vi "Sort Section Nodes.vi"(8 "error in":errorcluster, 10 "Nested Section Types":cluster{"Nested Section Types":string[]}[](array[cluster]), 11 "Section TypeNames":string[](array[string])) -> (0 "error out":errorcluster, 3 "Sorted Section TypeNames":string[](array[string]))   [LabVIEW 2026, in "Plugin XML Parser.lvlib"]
uses:
  Plugin XML Parser.lvlib
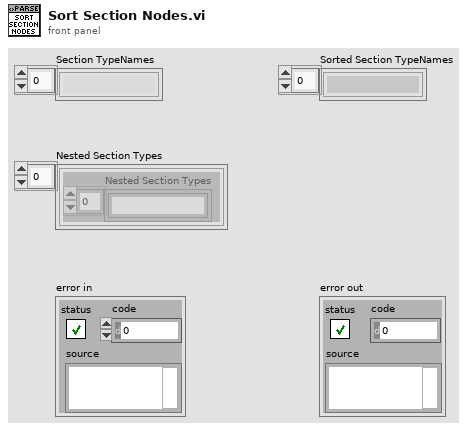
[diagram p1: front panel]
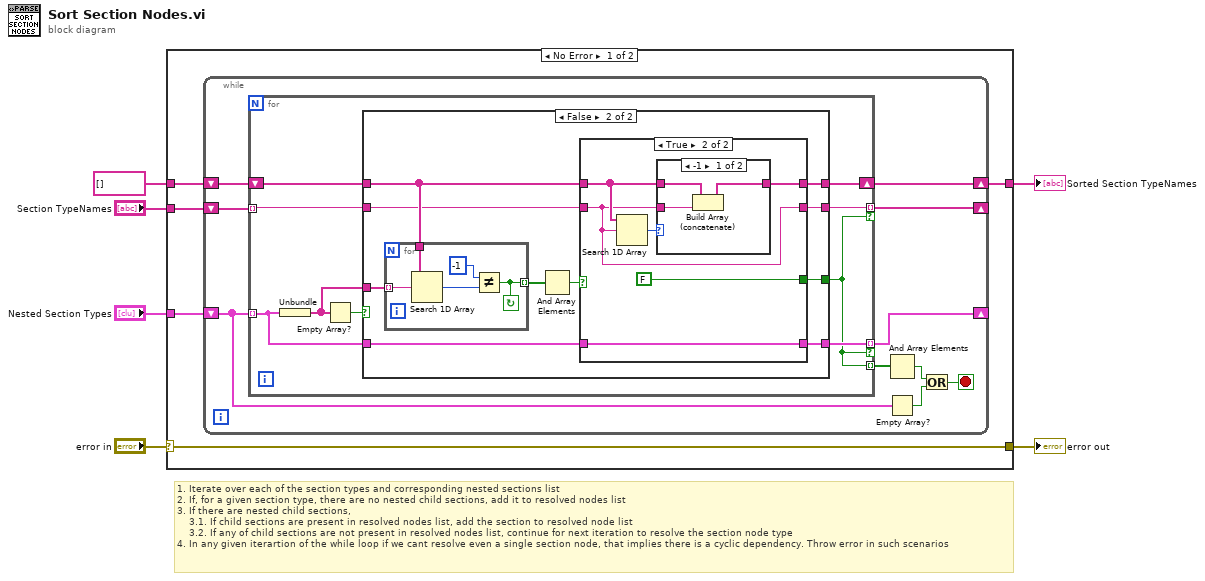
[diagram p0: block diagram]
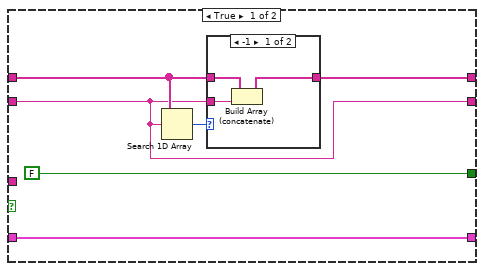
[diagram p2: hidden frame]
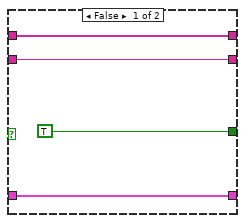
[diagram p4: hidden frame]
diagram:
  # "1. Iterate over each of the section types and corresponding nested sections list\n2. If, for a given section type, there are no nested child sections, add it to resolved nodes list\n3. If there are nested child sections,\n    3.1. If child sections are present in resolved nodes list, add the section to resolved node list\n    3.2. If any of child sections are not present in resolved nodes list, continue for next iteration to resolve the section node type\n4. In any given iterartion of the while loop if we cant resolve even a single section node, that implies there is a cyclic dependency. Throw error in such scenarios"
  n1 = case shown="No Error" "error in" {
    selector: "error in" -> [w7 w71]
    tunnel: string[] [] -> [w11 w70]
    tunnel: "Section TypeNames" -> [w10 _]
    tunnel: "Nested Section Types" -> [w9 _]
    tunnel: [w8 w70] -> w1
    tunnel: [w7 w71] -> w6
    frame No Error {
      n2 = while {
        shift-right: [w17] -> _
        shift-left: w10 -> [w18]
        shift-right: [w16] -> _
        shift-left: w9 -> [w15]
        shift-right: [w20] -> w8
        shift-left: w11 -> [w21]
        stop <- w13 stop-if-true
        n3 = for {
          tunnel: w18 -> [w30] mode=indexing
          tunnel: w15 -> [w23] mode=indexing
          shift-right: [w28] -> w20
          shift-left: w21 -> [w29]
          tunnel: [w22] -> w19 mode=indexing
          tunnel: [w26] -> w17 mode=indexing if=w22
          tunnel: [w25] -> w16 mode=indexing if=w22
          n4 = Unbundle(w23) -> ("Nested Section Types"=w24:string[])
          n5 = Empty Array?(array=w24) -> (empty?=w27:bool)
          n6 = case shown="False" w27 {
            tunnel: [w35 w50] -> w28
            tunnel: w30 -> [w33 w46]
            tunnel: w29 -> [w36 w47]
            tunnel: [w33 w49] -> w26
            tunnel: [w32 w48] -> w25
            tunnel: w24 -> [_ w43]
            tunnel: [FALSE w42] -> w22
            tunnel: w23 -> [w32 w41]
            frame True {
              n7 = Search 1D Array(1D array=w36, element=w33) -> (index of element=w31:i32)  [unwired: 1 in]
              n8 = case shown="-1" w31 {
                tunnel: [w39 w40] -> w35
                tunnel: w36 -> [w38 w40]
                tunnel: w33 -> [w37 _]
                frame -1 {
                  n9 = Build Array (concatenate)(w38, w37) -> (w39:string[])
                }
                frame 1, Default {
                }
              }
            }
            frame False {
              n10 = for {
                tunnel: w47 -> [w55]
                tunnel: [w51] -> w45 mode=indexing
                tunnel: w43 -> [w52] mode=indexing
                stop <- w51 continue-if-true
                n11 = Search 1D Array(1D array=w55, element=w52) -> (index of element=w54:i32)  [unwired: 1 in]
                n12 = Not Equal?(x=-1, y=w54) -> (x != y?=w51:bool)
              }
              n13 = And Array Elements(Boolean array=w45) -> (logical AND=w44:bool)
              n14 = case shown="True" w44 {
                tunnel: w46 -> [w56 w62]
                tunnel: [w59 w65] -> w50
                tunnel: w47 -> [w59 w64]
                tunnel: [w56 w62] -> w49
                tunnel: w41 -> [w58 w61]
                tunnel: [w58 w61] -> w48
                tunnel: [TRUE FALSE] -> w42
                frame False {
                }
                frame True {
                  n15 = Search 1D Array(1D array=w64, element=w62) -> (index of element=w60:i32)  [unwired: 1 in]
                  n16 = case shown="-1" w60 {
                    tunnel: [w68 w69] -> w65
                    tunnel: w64 -> [w67 w69]
                    tunnel: w62 -> [w66 _]
                    frame -1 {
                      n17 = Build Array (concatenate)(w67, w66) -> (w68:string[])
                    }
                    frame 1, Default {
                    }
                  }
                }
              }
            }
          }
        }
        n18 = And Array Elements(Boolean array=w19) -> (logical AND=w14:bool)
        n19 = Empty Array?(array=w15) -> (empty?=w12:bool)
        n20 = Or(x=w14, y=w12) -> (x .or. y?=w13:bool)
      }
    }
    frame Error {
    }
  }
  "Sorted Section TypeNames" <- w1
  "error out" <- w6
